vi "FINS out-read.vi"(8 "error i":errorcluster, 11 "FINS Header 2":T1 {"SNA" max=127 format="%x"; "SA2" max=254 step=1 format="%x"; "SA1" format="%x"; "DA2" max=254 step=1 format="%x"; "DA1" format="%x"; "DNA" max=127 step=1 format="%x"}) -> (0 "error o":errorcluster, 2 "msg":string, 3 "FINS Header":T1 {"SNA" max=127 format="%x"; "SA2" max=254 step=1 format="%x"; "SA1" format="%x"; "DA2" max=254 step=1 format="%x"; "DA1" format="%x"; "DNA" max=127 step=1 format="%x"})   [LabVIEW 2019]
uses:
  FINS/FINS_header.ctl
  FINS/FINS CMD item.ctl
  FINS/FINS TCP.lvlib
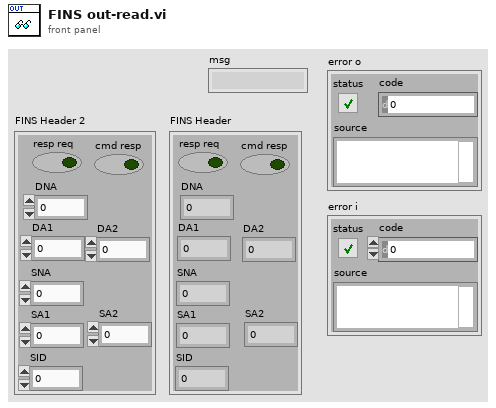
[diagram p1: front panel]
types:
  T1 = typedef "FINS TCP.lvlib/FINS_header.ctl" = cluster{"resp req":bool, "cmd resp":bool, "SID":u8, "DNA":u8, "DA1":u8, "DA2":u8, "SA1":u8, "SA2":u8, "SNA":u8}
  T2 = typedef "FINS TCP.lvlib/FINS CMD item.ctl" = enum16{"FINS_UNKNOWN", "FINS_SETUP", "MEMORY AREA READ", "MEMORY AREA WRITE", "MEMORY AREA FILL", "MULTIPLE MEMORY AREA READ", "MEMORY AREA TRANSFER", "PARAMETER AREA READ", "PARAMETER AREA WRITE", "PARAMETER AREA CLEAR", "PROGRAM AREA PROTECT", "PROGRAM AREA PROTECT CLEAR", "PROGRAM AREA READ", "PROGRAM AREA WRITE", "PROGRAM AREA CLEAR", "RUN", "STOP", "CONTROLLER DATA READ", "CONNECTION DATA READ", "CONTROLLER STATUS READ", "CYCLE TIME READ", "CLOCK READ", "CLOCK WRITE", "MESSAGE READ", "MESSAGE CLEAR", "FAL/FALS READ", "ACCESS RIGHT ACQUIRE", "ACCESS RIGHT FORCED ACQUIRE", "ACCESS RIGHT RELEASE", "ERROR CLEAR", "ERROR LOG READ", "ERROR LOG CLEAR", "FILE NAME READ", "SINGLE FILE READ", "SINGLE FILE WRITE", "MEMORY CARD FORMAT", "FILE DELETE", "VOLUME LABEL CREATE/DELETE", "FILE COPY", "FILE NAME CHANGE", "FILE DATA CHECK", "MEMORY AREA FILE TRANSFER", "PARAMETER AREA FILE TRANSFER", "PROGRAM AREA FILE TRANSFER", "FORCED SET/RESET", "FORCED SET/RESET CANCEL"}
  T3 = typedef "FINS TCP.lvlib/FINS CMD.ctl" = cluster{"MR":u8, "SR":u8, "name":string}
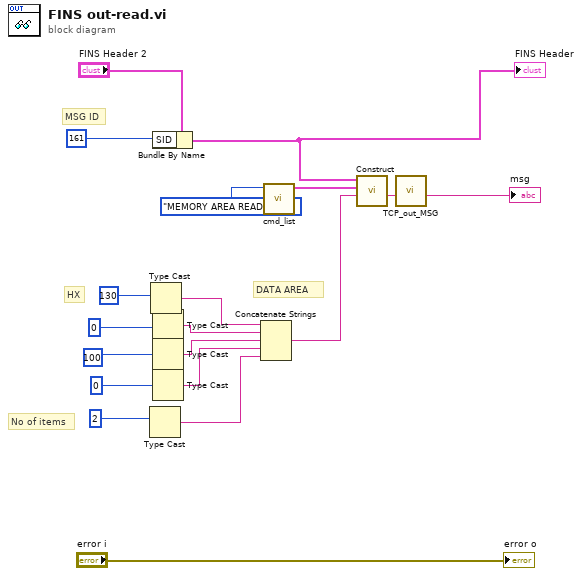
[diagram p0: block diagram]
diagram:
  # "No of items"
  # "DATA AREA"
  # "HX"
  # "MSG ID"
  n1 = Type Cast(x=u16 2 ("length")) -> (*(type *) &x=w8:string)  [unwired: 1 in]
  n2 = Type Cast(x=u8 130 ("length")) -> (*(type *) &x=w9:string)  [unwired: 1 in]
  n3 = Bundle By Name(cluster="FINS Header 2", "SID"=u8 161 ("SNA")) -> (w12:T1)
  "FINS Header" <- w12
  n4 = Type Cast(x=u8 0 ("length")) -> (*(type *) &x=w7:string)  [unwired: 1 in]
  n5 = Type Cast(x=u8 100 ("length")) -> (*(type *) &x=w6:string)  [unwired: 1 in]
  n6 = Type Cast(x=u8 0 ("length")) -> (*(type *) &x=w5:string)  [unwired: 1 in]
  n7 = Concatenate Strings(w9, w7, w6, w5, w8) -> (w1:string)
  n8 = call "cmd_list.vi"("CMD"=FINS_CMD_item."MEMORY AREA READ") -> ("cmd"=w17:T3)  [unwired: 9 in, 1 out]
  n9 = call "Construct.vi"("Paramters"=w1, "FINS CMD"=w17, "FINS Header"=w12) -> ("msg"=w19:string)  [unwired: 8 in]
  n10 = call "TCP_out_MSG.vi"("msgin"=w19) -> ("msg"=→"msg":string)  [unwired: 10 in]
  "error o" <- "error i"
